vi "CheckBox Callback.vi"(10 "Signal Parameter":i32, 11 "Receiver":refnum<class "LQObject.lvclass">) -> ()   [LabVIEW 2014, in "Dual Mode Thermometer.lvclass"]
doc: "Callback VI: Called when the user toggles the \"Farenheit\" checkbox.\n\n\nCopyright (c) 2019 Sze Howe Koh.\nThis code is licensed under the MIT license."
uses:
  Dual Mode Thermometer.lvclass
  <vilib>/addons/LQ/LQ Core/LQObject/LQObject.lvclass
  <vilib>/addons/LQ/LQ Core/Qt/CheckState.ctl
  Dual Mode Thermometer.lvclass/Dual Mode Thermometer.ctl
  <vilib>/addons/LQ/LQ Core/Qt/Qt.lvlib
  <vilib>/addons/LQ/Qwt/QwtAbstractSlider/QwtAbstractSlider.lvclass
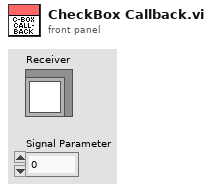
[diagram p1: front panel]
types:
  T1 = typedef "Qt.lvlib/CheckState.ctl" = i32
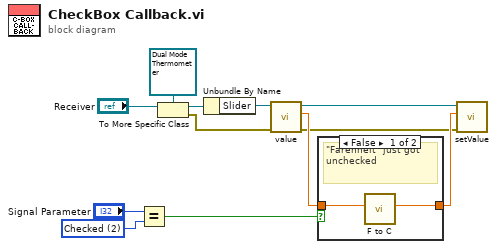
[diagram p0: block diagram]
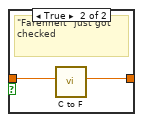
[diagram p2: hidden frame]
diagram:
  w7 = T1 2 items=["Unchecked", "PartiallyChecked", "Checked"] ("CheckState")
  n1 = Equal?(x="Signal Parameter", y=w7) -> (x = y?=w6:bool)
  n2 = To More Specific Class(target class=refnum<class "Dual Mode Thermometer.lvclass"> refnum ("Dual Mode Thermometer"), reference="Receiver") -> (specific class reference=w9:refnum<class "Dual Mode Thermometer.lvclass">, error out=w1:errorcluster)  [unwired: 1 in]
  n3 = Unbundle By Name(w9) -> ("Slider"=w12:refnum<class "QwtSlider.lvclass">)
  n4 = call <vilib>:"value.vi"("Error In"=w1, "QwtAbstractSlider In"=w12) -> ("Error Out"=w2:errorcluster, "Value"=w5:dbl, "QwtAbstractSlider Out"=w3:refnum<class "QwtSlider.lvclass">)  [unwired: 7 in]
  n5 = case shown="False" w6 {
    tunnel: w5 -> [w14 w16]
    tunnel: [w13 w15] -> w4
    frame False {
      # "\"Farenheit\" just got\nunchecked"
      n6 = call "F to C.vi"("Value [°F]"=w14) -> ("Value [°C]"=w13:dbl)  [unwired: 10 in]
    }
    frame True {
      # "\"Farenheit\" just got\nchecked"
      n7 = call "C to F.vi"("Value [°C]"=w16) -> ("Value [°F]"=w15:dbl)  [unwired: 10 in]
    }
  }
  n8 = call <vilib>:"setValue.vi"("Error In"=w2, "val"=w4, "QwtAbstractSlider In"=w3) -> ()  [unwired: 7 in, 2 out]
